vi "rangelimited.vi"(9 "Upper lim":fxp<+/-,32,16>, 10 "Input":fxp<+/-,32,16>, 11 "Lower lim":fxp<+/-,32,16>) -> (3 "Output":fxp<+/-,32,16>)   [LabVIEW 2012]
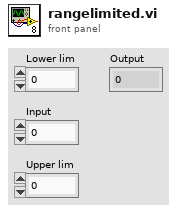
[diagram p1: front panel]
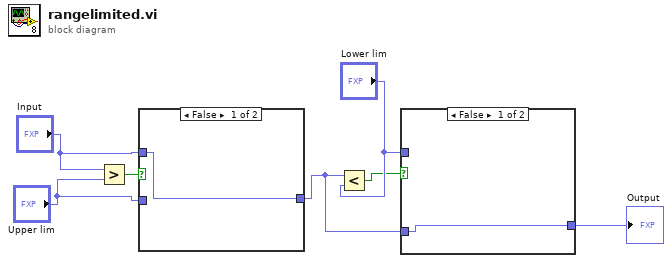
[diagram p0: block diagram]
diagram:
  n1 = Greater?(x="Input", y="Upper lim") -> (0:w1:bool)
  n2 = case shown="False" w1 {
    tunnel: "Upper lim" -> [_ w9]
    tunnel: [w8 w9] -> w7
    tunnel: "Input" -> [w8 _]
    frame False {
    }
    frame True {
    }
  }
  n3 = Less?(x=w7, y="Lower lim") -> (x < y?=w4:bool)
  n4 = case shown="False" w4 {
    tunnel: "Lower lim" -> [_ w11]
    tunnel: [w10 w11] -> w6
    tunnel: w7 -> [w10 _]
    frame False {
    }
    frame True {
    }
  }
  "Output" <- w6
